vi "Rectangle.vi"(10 "Heigth":dbl, 11 "Width":dbl) -> (3 "Rectangle Out":refnum<class "Rectangle.lvclass">)   [LabVIEW 2018, in "Rectangle.lvclass"]
uses:
  Rectangle.lvclass
  Rectangle.lvclass/Rectangle.ctl
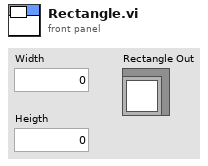
[diagram p1: front panel]
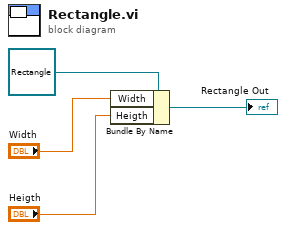
[diagram p0: block diagram]
diagram:
  n1 = Bundle By Name(cluster=refnum<class "Rectangle.lvclass"> refnum ("Rectangle in"), "Width"="Width", "Heigth"="Heigth") -> (→"Rectangle Out":refnum<class "Rectangle.lvclass">)
